vi "FrontPanelReferences.vi"() -> ()   [LabVIEW 2017, in "WaveformGenerator.lvlib"]
uses:
  WaveformGeneratorInterfaceRef.ctl
  WaveformGenerator.lvlib
panel:
  in  "References":T1
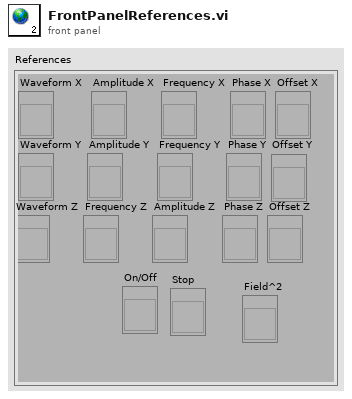
[diagram p1: front panel]
types:
  T1 = typedef "WaveformGenerator.lvlib/WaveformGeneratorInterfaceRef.ctl" = cluster{"Waveform X":refnum<vi>, "Waveform Y":refnum<vi>, "Waveform Z":refnum<vi>, "Amplitude X":refnum<vi>, "Amplitude Y":refnum<vi>, "Amplitude Z":refnum<vi>, "Frequency X":refnum<vi>, "Frequency Y":refnum<vi>, "Frequency Z":refnum<vi>, "Phase X":refnum<vi>, "Phase Y":refnum<vi>, "Phase Z":refnum<vi>, "Offset X":refnum<vi>, "Offset Y":refnum<vi>, "Offset Z":refnum<vi>, "Stop":refnum<vi>, "On/Off":refnum<vi>, "Field^2":refnum<vi>}
diagram:
